vi "MappingFunc(XYIntercept) (2).vi"(7 "Input":dbl format="%#_13g", 10 "Cluster":T1) -> (3 "Output":dbl)   [LabVIEW 2016]
panel:
  out "XY Graph":cluster{dbl[], dbl[]}(graph)
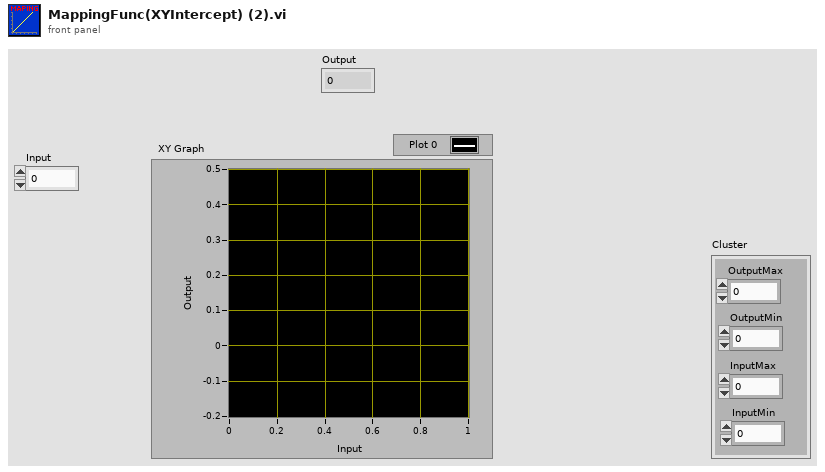
[diagram p1: front panel]
types:
  T1 = cluster{"OutputMax":dbl, "OutputMin":dbl, "InputMax":dbl, "InputMin":dbl}
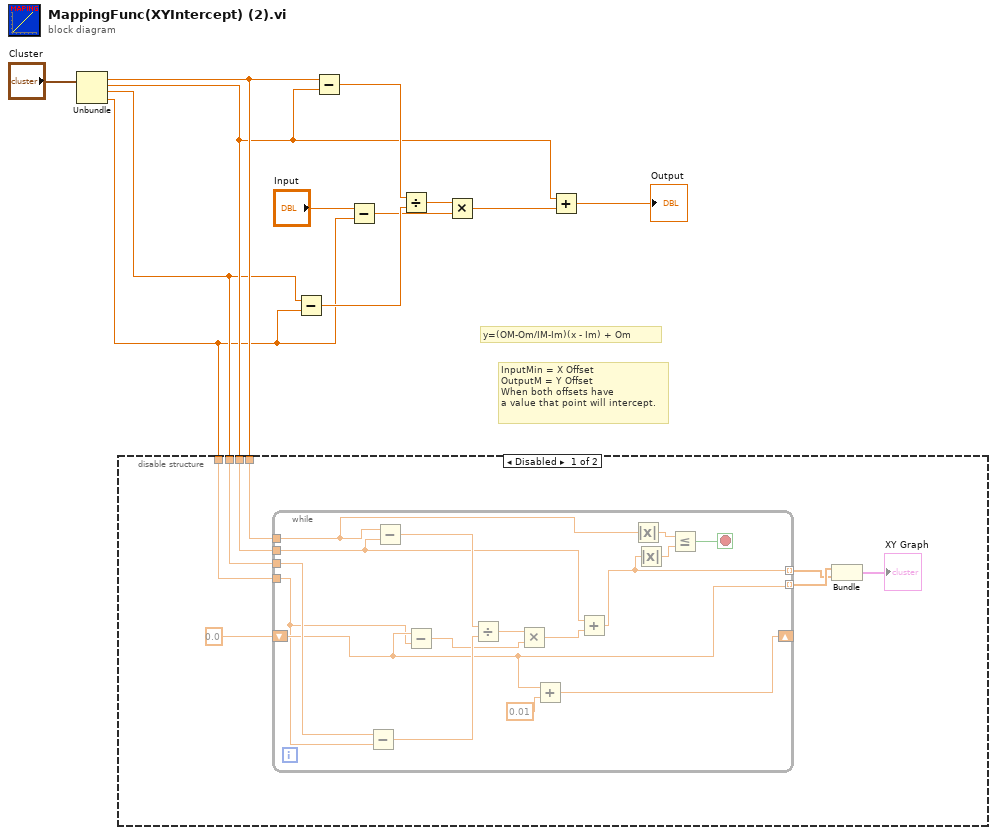
[diagram p0: block diagram]
diagram:
  # "InputMin = X Offset\nOutputM = Y Offset\nWhen both offsets have\na value that point will intercept."
  # "y=(OM-Om/IM-Im)(x - Im) + Om"
  n1 = Unbundle("Cluster") -> ("OutputMax"=w5:dbl, "OutputMin"=w3:dbl, "InputMax"=w2:dbl, "InputMin"=w1:dbl)
  n2 = disable-structure shown="Disabled" {
    disable-tunnel: w5 -> [w20 _]
    disable-tunnel: w3 -> [w19 _]
    disable-tunnel: w2 -> [w18 _]
    disable-tunnel: w1 -> [w17 _]
    frame Disabled {
      n3 = while {
        tunnel: w20 -> [w24]
        tunnel: w19 -> [w21]
        tunnel: w18 -> [w33]
        tunnel: w17 -> [w28]
        shift-right: [w31] -> _
        shift-left: 0.0 -> [w30]
        tunnel: [w30] -> w15 mode=indexing
        tunnel: [w22] -> w14 mode=indexing
        stop <- w27 stop-if-true
        n4 = Subtract(x=w33, y=w28) -> (x-y=w35:dbl)
        n5 = Subtract(x=w24, y=w21) -> (x-y=w36:dbl)
        n6 = Subtract(x=w30, y=w28) -> (x-y=w29:dbl)
        n7 = Divide(x=w36, y=w35) -> (x/y=w34:dbl)
        n8 = Multiply(x=w34, y=w29) -> (x*y=w23:dbl)
        n9 = Add(x=w30, y=0.01) -> (x+y=w31:dbl)
        n10 = Add(x=w21, y=w23) -> (x+y=w22:dbl)
        n11 = Absolute Value(x=w24) -> (abs(x)=w25:dbl)
        n12 = Absolute Value(x=w22) -> (abs(x)=w26:dbl)
        n13 = Less Or Equal?(x=w25, y=w26) -> (x <= y?=w27:bool)
      }
      n14 = Bundle(w15, w14) -> (→"XY Graph":cluster{dbl[], dbl[]})  [unwired: 1 in]
    }
    frame Enabled {
    }
  }
  n15 = Subtract(x=w2, y=w1) -> (x-y=w11:dbl)
  n16 = Subtract(x=w5, y=w3) -> (x-y=w12:dbl)
  n17 = Subtract(x="Input", y=w1) -> (x-y=w8:dbl)
  n18 = Divide(x=w12, y=w11) -> (x/y=w10:dbl)
  n19 = Multiply(x=w10, y=w8) -> (x*y=w6:dbl)
  n20 = Add(x=w3, y=w6) -> (x+y=→"Output":dbl)
